vi "SwapIntoArray.vi"(7 "enq":bool, 8 "element in":T1, 9 "last id":u32, 10 "index":i32, 11 "SubChannel in":refnum<class "SubChannelCPU.lvclass">) -> (0 "element out":T1, 1 "id":u32, 3 "SubChannel out":refnum<class "SubChannelCPU.lvclass">)   [LabVIEW 2019, in "MessengerM.lvlib" / "SubChannelCPU.lvclass"]
uses:
  SubChannelCPU.lvclass
  Element.ctl
  MessengerM.lvlib
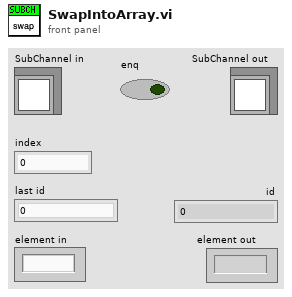
[diagram p1: front panel]
types:
  T1 = typedef "MessengerM.lvlib/Element.ctl" = string
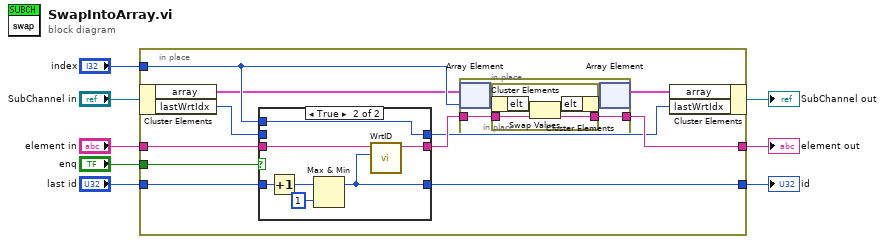
[diagram p0: block diagram]
diagram:
  n1 = in-place {
    in-place-border: [w19] -> w1
    in-place-border: "enq" -> [w18]
    in-place-border: "element in" -> [w17]
    in-place-border: "index" -> [w15]
    in-place-border: "last id" -> [w14]
    in-place-border: [w13] -> w2
    n2 = in-place-cluster #1("SubChannel in") -> ("array"=w10:cluster{"elt":T1}[], "lastWrtIdx"=w12:i32)
    n3 = case shown="True" w18 {
      tunnel: w17 -> [w21 w25]
      tunnel: [w21 w24] -> w16
      tunnel: w14 -> [w22 w29]
      tunnel: [w22 w23] -> w13
      tunnel: [w20 w26] -> w11
      tunnel: w12 -> [w20 _]
      tunnel: w15 -> [_ w26]
      frame False {
      }
      frame True {
        n4 = Increment(x=w29) -> (x+1=w28:u32)
        n5 = Max & Min(x=w28, y=u32 1) -> (max(x,y)=w23:u32)  [unwired: 1 out]
        n6 = call "WrtID.vi"("id"=w23, "element in"=w25) -> ("element out"=w24:T1)  [unwired: 9 in]
      }
    }
    n7 = in-place {
      in-place-border: w16 -> [w33]
      in-place-border: [w32] -> w19
      n8 = in-place-array #2(w10, w15) -> (w31:cluster{"elt":T1})
      n9 = in-place {
        in-place-border: w33 -> [w37]
        in-place-border: [w36] -> w32
        n10 = in-place-cluster #3(w31) -> ("elt"=w35:T1)
        n11 = Swap Values(12:w35, 14:w37) -> (1:w34:T1, 3:w36:T1)  [unwired: 1 in]
        n12 = in-place-cluster #3("elt"=w34) -> (w30:cluster{"elt":T1})
      }
      n13 = in-place-array #2(w30) -> (w9:cluster{"elt":T1}[])  [unwired: 1 out]
    }
    n14 = in-place-cluster #1("array"=w9, "lastWrtIdx"=w11) -> (→"SubChannel out":refnum<class "SubChannelCPU.lvclass">)
  }
  "element out" <- w1
  "id" <- w2
